vi "Main Global.vi"() -> ()   [LabVIEW 2010]
uses:
  Streaming Data.ctl
  UART/UART Port Type.ctl
panel:
  in  "VISA resource name":T1="COM5"
  in  "Spin Right?":bool
  in  "Drive Speed":dbl
  in  "Drive Radius":dbl
  in  "Angle Update in degrees":i16
  in  "Distance Update in mm":i16
  in  "Y Coordinate":dbl
  in  "X Coordinate":dbl
  in  "Pose in Radians":dbl
  out "Streaming Data":T2
  # "dictOut['Bump Right']=data[1]&0x01\n    dictOut['Bump Left']=(data[1]&0x02)>>1\n    dictOut['Wheeldrop Right']=(data[1]&0x04)>>2\n    dictOut['Wheeldrop Left']=(data[1]&0x08)>>3\n    dictOut['Wheeldrop Caster']=(data[1]&0x10)>>4\n    dictOut['Wall']=data[3]&0x01\n    dictOut['Cliff Left']=data[5]&0x01\n    dictOut['Cliff Front Left']=data[7]&0x01\n    dictOut['Cliff Front Right']=data[9]&0x01\n    dictOut['Cliff Right']=data[11]&0x01\n    IRdict={255:[0,0,0],168:[1,0,0],164:[0,1,0],161:[0,0,1],172:[1,1,0],169:[1,0,1],165:[0,1,1],173:[1,1,1]}\n    dictOut['IR Red']=IRdict[data[13]][0]\n    dictOut['IR Green']=IRdict[data[13]][1]\n    dictOut['IR Force']=IRdict[data[13]][2]\n    dictOut['Button Play']=data[15]&0x01\n    dictOut['Button Advance']=(data[15]&0x04)>>2\n    dictOut['Battery Charge']=data[17]"
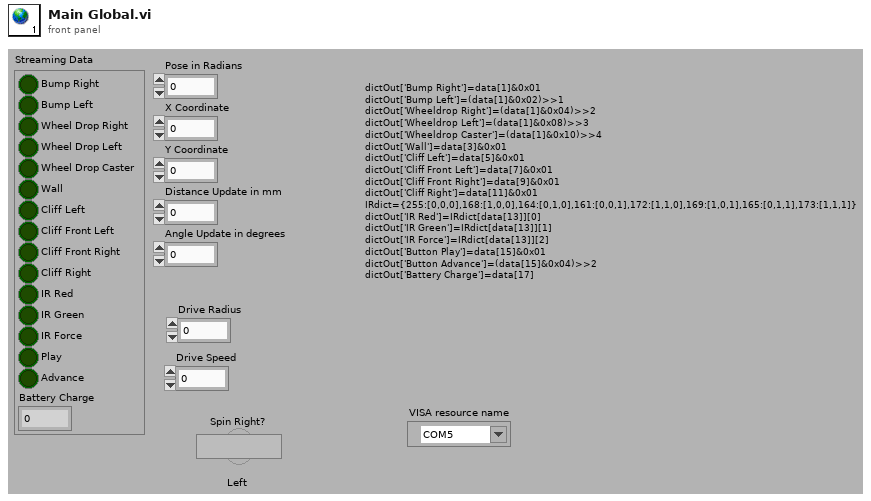
[diagram p1: front panel]
types:
  T1 = typedef "UART Port Type.ctl" = refnum<visa-resource-name>
  T2 = typedef "Streaming Data.ctl" = cluster{"Bump Right":bool, "Bump Left":bool, "Wheel Drop Right":bool, "Wheel Drop Left":bool, "Wheel Drop Caster":bool, "Wall":bool, "Cliff Left":bool, "Cliff Front Left":bool, "Cliff Front Right":bool, "Cliff Right":bool, "IR Red":bool, "IR Green":bool, "IR Force":bool, "Play":bool, "Advance":bool, "Battery Charge":i16}
diagram:
